vi "Gserver_X_constraints_request.vi"(8 "error in (no error)":errorcluster, 10 "Requester":string, 11 "FAMM in":refnum<class "FAMM.lvclass">) -> (0 "error out":errorcluster, 3 "FAMM out":refnum<class "FAMM.lvclass">)   [LabVIEW 2020]
doc: "Andre Koelewijn, 17 jan 2021\n\nThis VI will process a query as received from Gserver,\nthis query is a request for one of the Gviewer instances."
uses:
  FAMM.lvclass
  Gserver/controls/Typedef_QueryType.ctl
  controls/FAMM_reply_X_constraints.ctl
  Gserver/Gserver.lvclass
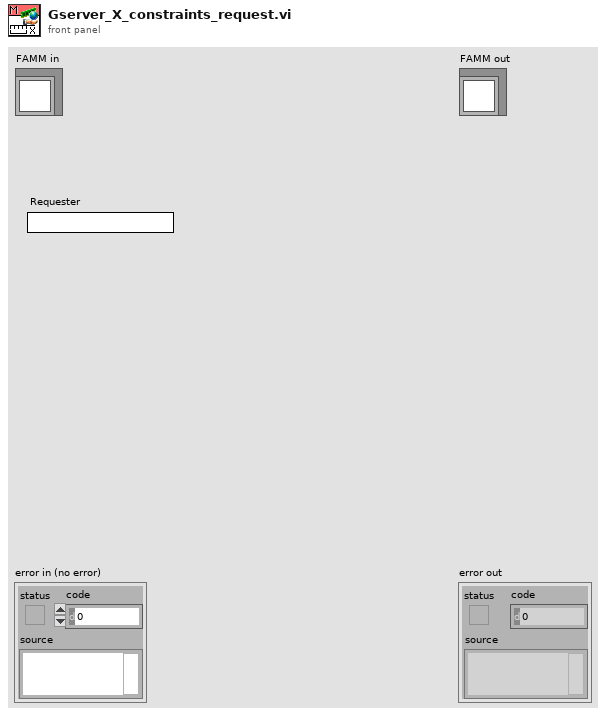
[diagram p1: front panel]
types:
  T1 = typedef "FAMM_reply_X_constraints.ctl" = cluster{"GraphName":string, "FAMM_PAQ_resolution":dbl, "data-retention(days)":dbl}
  T2 = typedef "Sgraph_lib_V1.lvlib/Gserver.lvclass/Typedef_QueryType.ctl" = enum16{"Subscribe", "DataRequest", "RequestAllTags", "RequestIniPath", "FAMMstarted", "SetClientOptions", "GviewerUpdate", "OpenNewGraph", "CloseClient", "CloseAllClients", "Close Gserver", "OpenMemoryMap", "MeMapDataRequest", "MeMapDataResponse", "OpenDBeditor", "CheckDBeditorRunning", "StoppedDBeditor", "SaveDB_TAGpropRecord", "ConfirmDB_TAGpropSave", "ReturnXconstraints"}
  T3 = cluster{"FAMM_PAQ_resolution":dbl, "data-retention(days)":dbl}
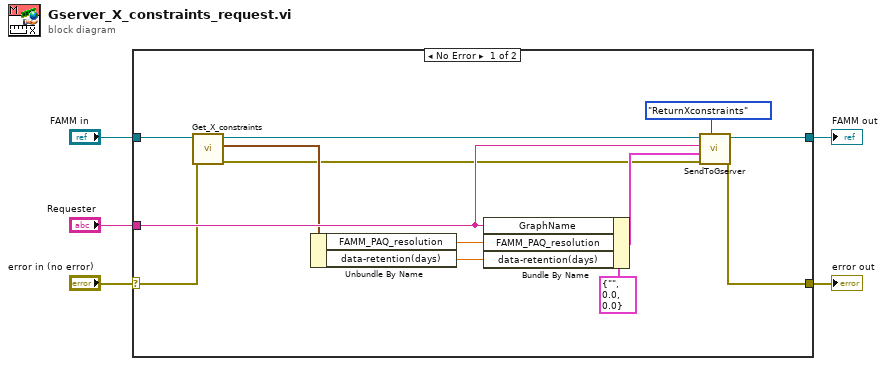
[diagram p0: block diagram]
diagram:
  n1 = case shown="No Error" "error in (no error)" {
    selector: "error in (no error)" -> [w7 w20]
    tunnel: [w17 w20] -> w4
    tunnel: [w18 w19] -> w2
    tunnel: "FAMM in" -> [w11 w19]
    tunnel: "Requester" -> [w16 _]
    frame No Error {
      n2 = call-dynamic "Get_X_constraints.vi"("error in (no error)"=w7, "FAMM in"=w11) -> ("error out"=w6:errorcluster, "X-constraints"=w10:T3, "FAMM out"=w12:refnum<class "FAMM.lvclass">)  [unwired: 7 in]
      n3 = Unbundle By Name(w10) -> ("FAMM_PAQ_resolution"=w9:dbl, "data-retention(days)"=w8:dbl)
      n4 = Bundle By Name(cluster=T1 {"GraphName"="", "FAMM_PAQ_resolution"=0.0, "data-retention(days)"=0.0} ("GviewerUpdate"), "GraphName"=w16, "FAMM_PAQ_resolution"=w9, "data-retention(days)"=w8) -> (w15:T1)
      n5 = call "SendToGserver.vi"("Query_type"=Typedef_QueryType."ReturnXconstraints", "error in (no error)"=w6, "data"=w15, "Address"=w16, "FAMM in"=w12) -> ("error out"=w17:errorcluster, "FAMM out"=w18:refnum<class "FAMM.lvclass">)  [unwired: 5 in]
    }
    frame Error {
    }
  }
  "error out" <- w4
  "FAMM out" <- w2
